vi "pcfs_write_pcfs_settings.vi"(8 "error in (no error)":errorcluster, 10 "pcfs_settings":T1={"Center Pos. (mm)"=0.0, "Increment (mm)"=0.0, "Steps"=0.0, "Dither Dist (nm)"=0.0, "Dither Period (s)"=0.0, "Cycles"=0.0, "Record Type"=enum."hdf5", "Save Path"=path "", "Stage Number"=enum."1", "File Notes"="", "Mode"=2, "overwrite"=FALSE, "custom_path"=FALSE, "custom_positions"=[]} {"Mode" items=["T2"=2, "T3"=3]}, 11 "pcfs in":refnum<class "pcfs.lvclass">) -> (0 "error out":errorcluster, 3 "pcfs out":refnum<class "pcfs.lvclass">)   [LabVIEW 2015, in "pcfs.lvclass"]
uses:
  pcfs.lvclass
  pcfs_settings.ctl
  Scan/scan_record.ctl
  Detector_Class/Picoquant/Hydraharp/hydraharp_panel/hpanel_acq_modes.ctl
  pcfs_position_settings.ctl
  Stage Class/Newport XPS/newport_xps/dither_trajectory_settings.ctl
  Stage Class/Newport XPS/newport_xps/dither_trajectory_types.ctl
  pcfs.lvclass/pcfs.ctl
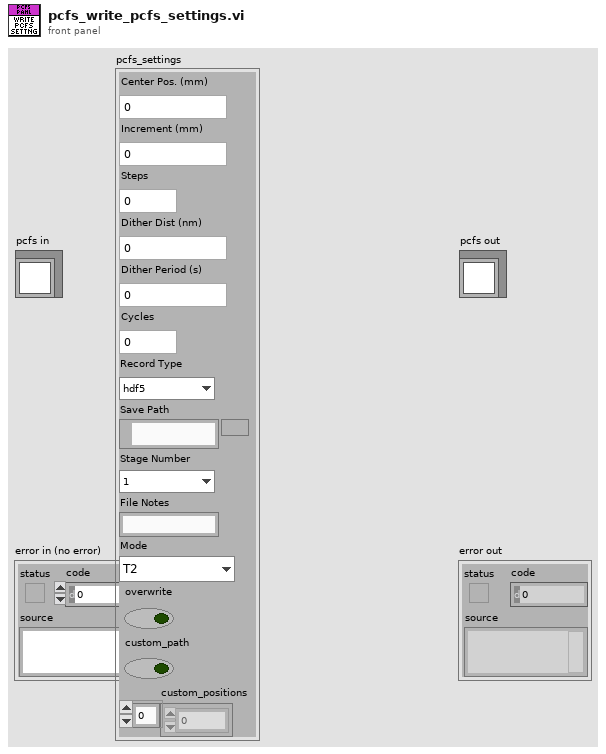
[diagram p1: front panel]
types:
  T1 = typedef "pcfs_settings.ctl" = cluster{"Center Pos. (mm)":dbl, "Increment (mm)":dbl, "Steps":dbl, "Dither Dist (nm)":dbl, "Dither Period (s)":dbl, "Cycles":dbl, "Record Type":T2, "Save Path":path, "Stage Number":enum16{"1", "2"}, "File Notes":string, "Mode":T3, "overwrite":bool, "custom_path":bool, "custom_positions":dbl[]}
  T2 = typedef "scan_record.ctl" = enum16{"hdf5", "legacy", "None"}
  T3 = typedef "hpanel_acq_modes.ctl" = u16
  T4 = typedef "dither_trajectory_types.ctl" = enum16{"Sawtooth"}
  T5 = typedef "dither_trajectory_settings.ctl" = cluster{"PVT Ampl (nm)":dbl, "Dither Period (s)":dbl, "Type":T4, "Name":string}
  T6 = typedef "pcfs_position_settings.ctl" = cluster{"Center Pos. (mm)":dbl, "increment":dbl, "steps":dbl, "dither_dist":dbl, "dither_period":dbl}
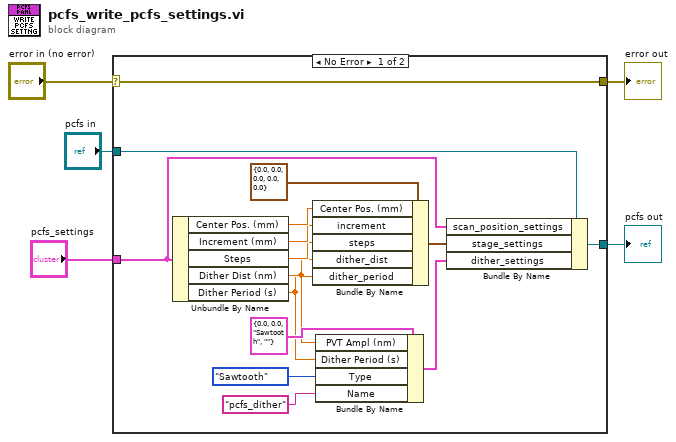
[diagram p0: block diagram]
diagram:
  n1 = case shown="No Error" "error in (no error)" {
    selector: "error in (no error)" -> [w20 w22]
    tunnel: [w20 w22] -> w4
    tunnel: [w12 w21] -> w2
    tunnel: "pcfs in" -> [w15 w21]
    tunnel: "pcfs_settings" -> [w14 _]
    frame No Error {
      n2 = Unbundle By Name(w14) -> ("Center Pos. (mm)"=w18:dbl, "Increment (mm)"=w17:dbl, "Steps"=w16:dbl, "Dither Dist (nm)"=w10:dbl, "Dither Period (s)"=w9:dbl)
      n3 = Bundle By Name(cluster=T6 {"Center Pos. (mm)"=0.0, "increment"=0.0, "steps"=0.0, "dither_dist"=0.0, "dither_period"=0.0} ("output cluster"), "Center Pos. (mm)"=w18, "increment"=w17, "steps"=w16, "dither_dist"=w10, "dither_period"=w9) -> (w13:T6)
      n4 = Bundle By Name(cluster=T5 {"PVT Ampl (nm)"=0.0, "Dither Period (s)"=0.0, "Type"=enum."Sawtooth", "Name"=""} ("output cluster"), "PVT Ampl (nm)"=w10, "Dither Period (s)"=w9, "Type"=dither_trajectory_types."Sawtooth", "Name"="pcfs_dither") -> (w6:T5)
      n5 = Bundle By Name(cluster=w15, "scan_position_settings"=w14, "stage_settings"=w13, "dither_settings"=w6) -> (w12:refnum<class "pcfs.lvclass">)
    }
    frame Error {
    }
  }
  "error out" <- w4
  "pcfs out" <- w2
